vi "ASCII HEX TO SYMBOLS.vi"(1 "ASCII HEX":string) -> (0 "Symbol":string)   [LabVIEW 2017, in "LV_Unicorn.lvlib"]
uses:
  LV_Unicorn.lvlib
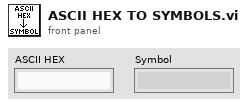
[diagram p1: front panel]
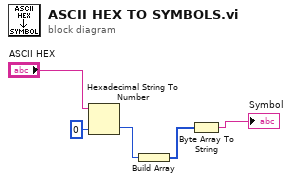
[diagram p0: block diagram]
diagram:
  n1 = Hexadecimal String To Number(string="ASCII HEX", default (0uL)=u8 0 ("default (0 U32)")) -> (number=w3:u8)  [unwired: 1 in, 1 out]
  n2 = Build Array(w3) -> (w2:u8[])
  n3 = Byte Array To String(unsigned byte array=w2) -> (string=→"Symbol":string)
